vi "processGObjects.vi"(8 "error in (no error)":errorcluster, 9 "Calling VI Reference i":refnum<vi>, 10 "All Objects[]":refnum<vi>[](array[refnum]), 11 "DiagramObject in":refnum<class "DiagramObject.lvclass">) -> (0 "error out":errorcluster, 3 "DiagramObject out":refnum<class "DiagramObject.lvclass">)   [LabVIEW 2016, in "DiagramObject.lvclass"]
uses:
  DiagramObject.lvclass
  DiagramObject.lvclass/DiagramObject.ctl
  Search/Search.lvclass/Search.ctl
  GObject/GObject.lvclass/GObject.ctl
  IGObjectFactory/IGObjectFactory.lvclass
  GObject/GObject.lvclass
  Project/Project.lvclass
  Search/Search.lvclass
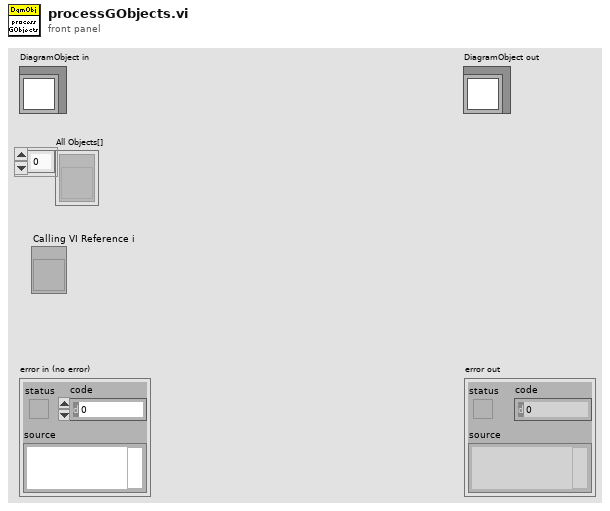
[diagram p1: front panel]
types:
  T1 = typedef "GObjectSelection.ctl" = enum16{"Default", "CaseStructure", "ClusterConstant", "EnumConstant", "EventStructure", "FlatSequence", "ForLoop", "WhileLoop"}
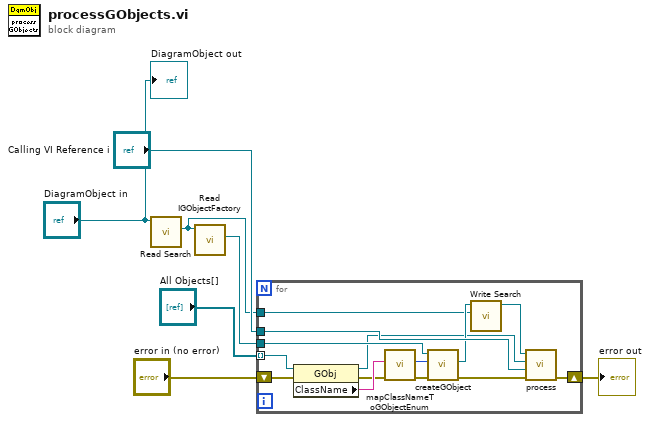
[diagram p0: block diagram]
diagram:
  n1 = call "Read Search.vi"("DiagramObject in"="DiagramObject in") -> ("Search"=w2:refnum<class "Search.lvclass">)  [unwired: 9 in, 1 out]
  n2 = call "Read IGObjectFactory.vi"("Search in"=w2) -> ("IGObjectFactory"=w1:refnum<class "IGObjectFactory.lvclass">)  [unwired: 9 in, 1 out]
  n3 = for {
    tunnel: "All Objects[]" -> [w19] mode=indexing
    tunnel: "Calling VI Reference i" -> [w18]
    shift-right: [w13] -> w4
    shift-left: "error in (no error)" -> [w17]
    tunnel: w2 -> [w10]
    tunnel: w1 -> [w9]
    n4 = property class="GObj"(reference=w19, error in=w17) -> (reference out=w8:refnum<vi>, error out=w16:errorcluster, "ClassName"=w21:string)
    n5 = call "mapClassNameToGObjectEnum.vi"("error in (no error)"=w16, "Class Name"=w21) -> ("error out"=w15:errorcluster, "GObjectSelection"=w20:T1)  [unwired: 7 in, 1 out]
    n6 = call-dynamic "createGObject.vi"("error in (no error)"=w15, "GObjectSelection"=w20, "IGObjectFactory in"=w9) -> ("error out"=w14:errorcluster, "GObject"=w12:refnum<class "GObject.lvclass">)  [unwired: 6 in, 1 out]
    n7 = call "Write Search.vi"("Search.lvclass"=w10, "DiagramObject in"=w12) -> ("DiagramObject out"=w11:refnum<class "GObject.lvclass">)  [unwired: 9 in]
    n8 = call-dynamic "process.vi"("error in (no error)"=w14, "Calling VI Reference i"=w18, "GObj Refnum"=w8, "DiagramObject in"=w11) -> ("error out"=w13:errorcluster)  [unwired: 6 in, 1 out]
  }
  "error out" <- w4
  "DiagramObject out" <- "DiagramObject in"
